vi "Configure Pattern Trigger.vi"(7 "Condition (True)":u32(slide) scale=0.0..5.0, 8 "error in (no error)":errorcluster {"code" format="%.0x"}, 9 "Delta Time (s)":dbl=0.01 format="%.2p", 10 "Function (0: AND)":i32(ring) items=["AND", "OR", "NAND", "NOR"], 11 "VISA Resource Name":refnum<visa-resource-name>) -> (0 "error out":errorcluster {"code" format="%.0x"}, 3 "VISA Resource Name Out":refnum<visa-resource-name>)   [LabVIEW 2010, in "Tektronix TDS 3000 Series.lvlib"]
doc: "This VI configures the pattern triggering. This enables pattern triggering, which triggers the oscilloscope when the logic condition (pattern) on two inputs is met.\n\nNotes:\n\n(1) This VI affects instrument behavior only if the Trigger Type is set to Pattern Trigger. Call the Configure Trigger VI to set the Trigger Type before you call this VI."
uses:
  <instrlib>/Tektronix TDS 3000 Series/Tektronix TDS 3000 Series.lvlib
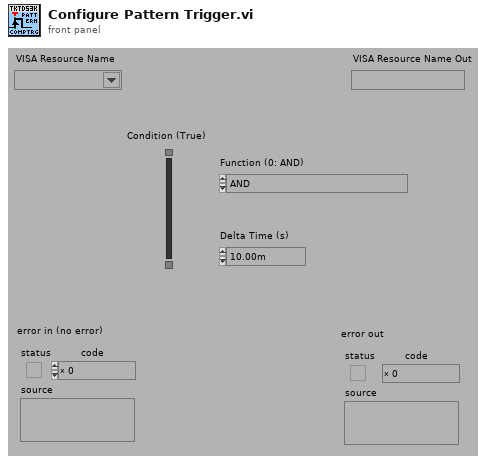
[diagram p1: front panel]
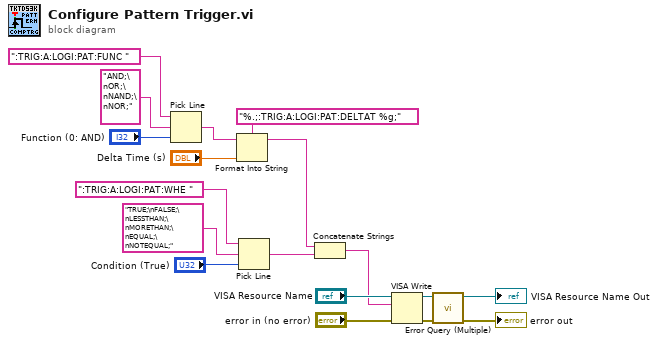
[diagram p0: block diagram]
diagram:
  n1 = Pick Line(string ("")=":TRIG:A:LOGI:PAT:FUNC ", multi-line string="AND;\nOR;\nNAND;\nNOR;", line index="Function (0: AND)") -> (output string=w13:string)
  n2 = Format Into String(format string="%.;:TRIG:A:LOGI:PAT:DELTAT %g;", initial string=w13, "Delta Time (s)") -> (resulting string=w6:string)  [unwired: 1 in, 1 out]
  n3 = Pick Line(string ("")=":TRIG:A:LOGI:PAT:WHE ", multi-line string="TRUE;\nFALSE;\nLESSTHAN;\nMORETHAN;\nEQUAL;\nNOTEQUAL;", line index="Condition (True)") -> (output string=w7:string)
  n4 = Concatenate Strings(w6, w7) -> (w5:string)
  n5 = VISA Write(VISA resource name="VISA Resource Name", write buffer=w5, error in (no error)="error in (no error)") -> (VISA resource name out=w4:refnum<visa-resource-name>, error out=w3:errorcluster)  [unwired: 1 out]
  n6 = call <instrlib>:"Error Query (Multiple).vi"("error in (no error)"=w3, "VISA Resource Name"=w4) -> ("error out"=→"error out":errorcluster, "VISA Resource Name Out"=→"VISA Resource Name Out":refnum<visa-resource-name>)  [unwired: 6 in, 2 out]
